vi "cDAQ Test.vi"() -> ()   [LabVIEW 2023]
panel:
  in  "milliseconds to wait":u32=1000
  out "Loop Index":i32=7776579
  in  "stop":bool
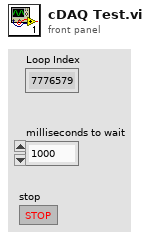
[diagram p1: front panel]
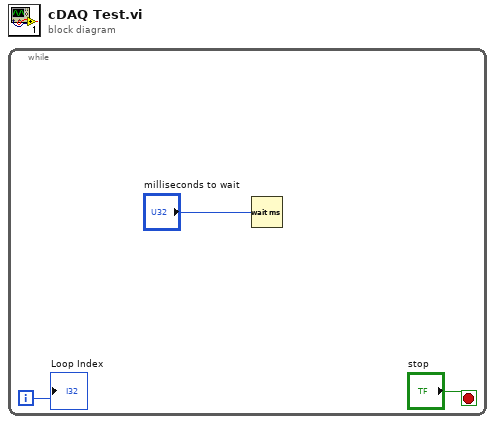
[diagram p0: block diagram]
diagram:
  n1 = while {
    i -> [w2]
    stop <- "stop" stop-if-true
    n2 = Wait (ms)(milliseconds to wait="milliseconds to wait") -> ()  [unwired: 1 out]
    "Loop Index" <- w2
  }
